vi "VariabilaGlobala.vi"() -> ()   [LabVIEW 2025]
panel:
  in  "RezultatPredictie":string[](array[string])
  out "HartaPixeli":bool[][](array[boolean])
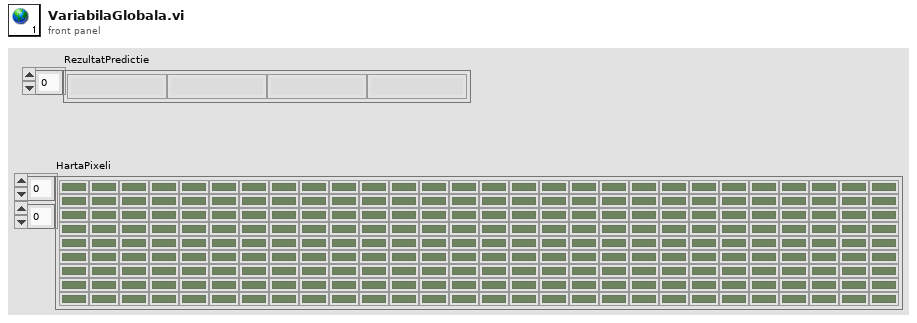
[diagram p1: front panel]
diagram:
